vi "Load PID from DB.vi"(8 "error in":errorcluster, 11 "Name":string="Numeric Array") -> (0 "error out":errorcluster, 2 "PID":T1)   [LabVIEW 2016]
uses:
  PID Settings.ctl
  <vilib>/Rock Robotics/Network Tables/NT Read Numeric Array.vi
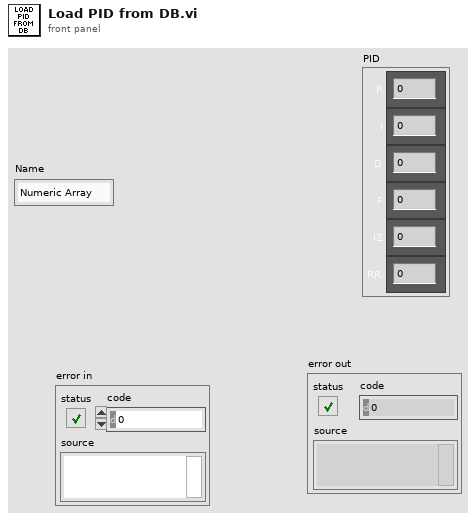
[diagram p1: front panel]
types:
  T1 = typedef "PID Settings.ctl" = cluster{"D":dbl, "F":dbl, "RR":dbl, "IZ":dbl, "P":dbl, "I":dbl}
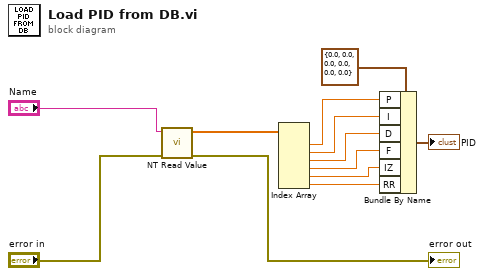
[diagram p0: block diagram]
diagram:
  n1 = call-poly <vilib>:"NT Read Value.vi"("error in"="error in", "Name"="Name") -> ("error out"=→"error out":errorcluster, "Numeric Array"=w11:dbl[])  [unwired: 8 in]
  n2 = Index Array(array=w11) -> (element #1=w9:dbl, element #2=w8:dbl, element #3=w7:dbl, element #4=w6:dbl, element #5=w5:dbl, element #6=w4:dbl)  [unwired: 6 in]
  n3 = Bundle By Name(cluster=T1 {"D"=0.0, "F"=0.0, "RR"=0.0, "IZ"=0.0, "P"=0.0, "I"=0.0} ("PID"), "P"=w9, "I"=w8, "D"=w7, "F"=w6, "IZ"=w5, "RR"=w4) -> (→"PID":T1)
